vi "trapezoidal_subvi.vi"(8 "frequency":i32(knob)=1 min=1 max=100 step=1 scale=0.0..100.0, 9 "Offset in":dbl, 10 "Amplitude in":dbl, 11 "number of cycles":dbl) -> (3 "Waveform Graph":waveform(dbl)(graph))   [LabVIEW 2020]
uses:
  <vilib>/Analysis/1siggen.llb/Ramp Pattern by Samples.vi
  <vilib>/Analysis/NI_AALBase.lvlib
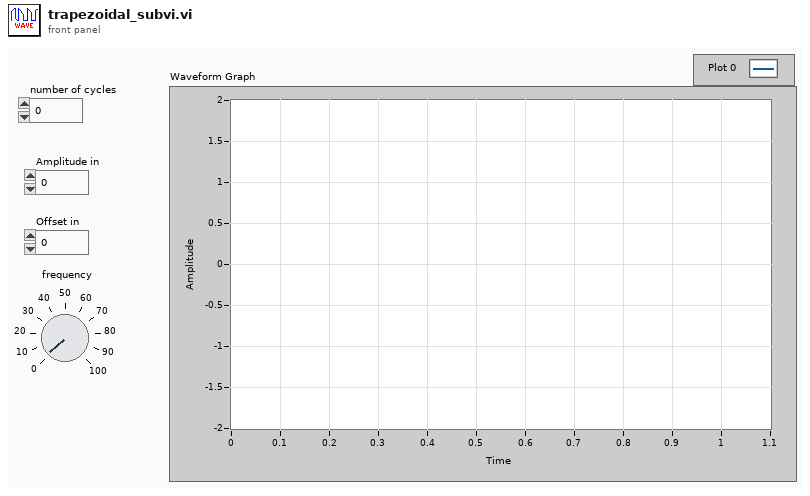
[diagram p1: front panel]
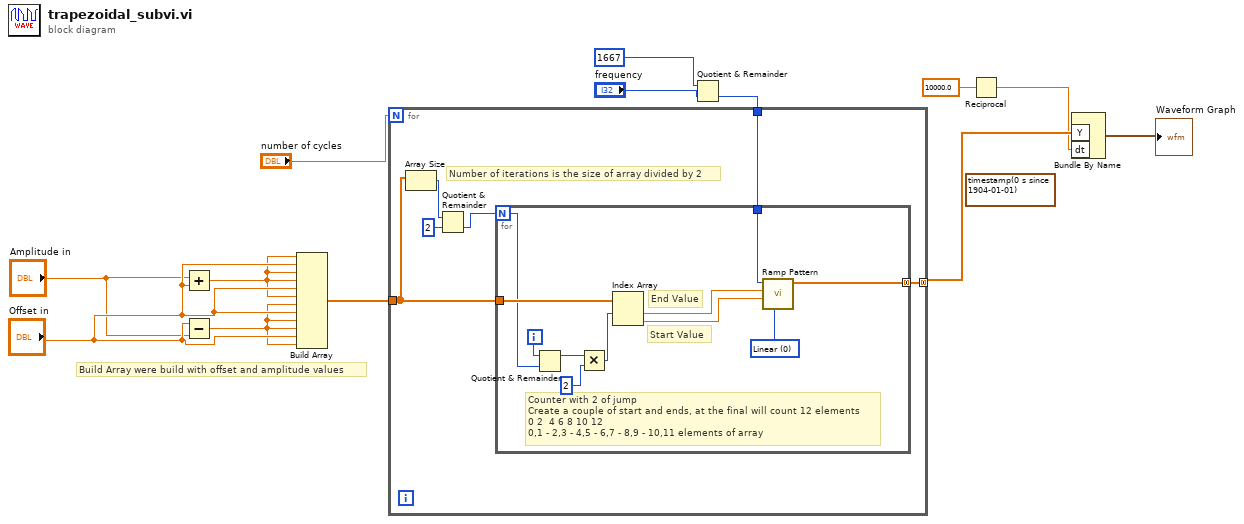
[diagram p0: block diagram]
diagram:
  (unwired) timestamp(0 s since 1904-01-01)
  # "Build Array were build with offset and amplitude values"
  n1 = Add(x="Amplitude in", y="Offset in") -> (x+y=w9:dbl)
  n2 = Subtract(x="Offset in", y="Amplitude in") -> (x-y=w10:dbl)
  n3 = Build Array(w9, "Offset in", w9, w9, "Offset in", w9, w10, "Offset in", w10, w10, "Offset in", w10) -> (w11:dbl[])
  n4 = Quotient & Remainder(x=1667, y="frequency") -> (floor(x/y)=w4:i32)  [unwired: 1 out]
  n5 = for {
    N: "number of cycles" -> [_]
    tunnel: [w19] -> w8 mode=concatenating
    tunnel: w11 -> [w18]
    tunnel: w4 -> [w14]
    # "Number of iterations is the size of array divided by 2"
    n6 = Array Size(array=w18) -> (size(s)=w17:i32)
    n7 = Quotient & Remainder(x=w17, y=2) -> (floor(x/y)=w15:i32)  [unwired: 1 out]
    n8 = for {
      N: w15 -> [w21]
      tunnel: w18 -> [w29]
      tunnel: [w26] -> w19 mode=concatenating
      tunnel: w14 -> [w20]
      i -> [w23]
      w30 = u16 0 items=["Linear", "Logarithmic"] ("type")
      # "End Value"
      # "Start Value"
      # "Counter with 2 of jump\nCreate a couple of start and ends, at the final will count 12 elements\n0 2  4 6 8 10 12\n0,1 - 2,3 - 4,5 - 6,7 - 8,9 - 10,11 elements of array"
      n9 = Quotient & Remainder(x=w23, y=w21) -> (x-y*floor(x/y)=w25:i32)  [unwired: 1 out]
      n10 = Multiply(x=w25, y=2) -> (x*y=w22:i32)
      n11 = Index Array(array=w29, index #1=w22) -> (element #1=w27:dbl, element #2=w28:dbl)  [unwired: 1 in]
      n12 = call-poly <vilib>:"Ramp Pattern.vi"("type"=w30, "start"=w28, "end"=w27, "samples"=w20) -> ("Ramp Pattern"=w26:dbl[])  [unwired: 6 in, 1 out]
    }
  }
  n13 = Reciprocal(x=10000.0) -> (1/x=w3:dbl)
  n14 = Bundle By Name("Y"=w8, "dt"=w3) -> (→"Waveform Graph":waveform(dbl))  [unwired: 1 in]
